vi "controlContinousBkwd.vi"(7 "Set":bool, 8 "error in":errorcluster, 9 "continous BWD in":bool=TRUE, 10 "axis in":u8, 11 "connection ID":i32) -> (0 "error out":errorcluster, 1 "continous BWD out":bool=TRUE, 2 "axis out":u8, 3 "connection ID":i32)   [LabVIEW 2016]
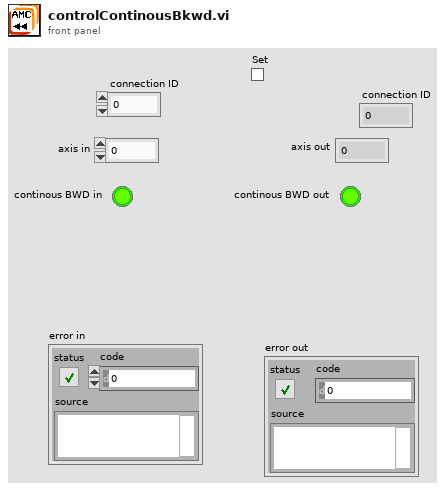
[diagram p1: front panel]
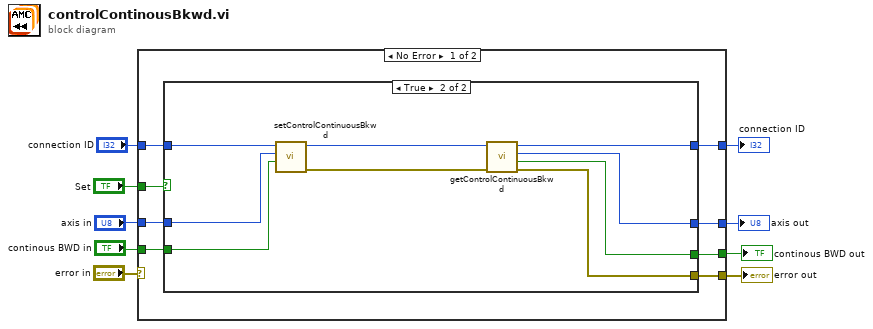
[diagram p0: block diagram]
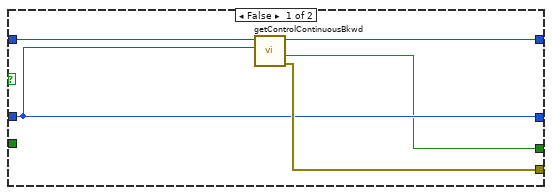
[diagram p2: hidden frame]
diagram:
  n1 = case shown="No Error" "error in" {
    selector: "error in" -> [_ w35]
    tunnel: "axis in" -> [w15 w33]
    tunnel: [w10 w35] -> w8
    tunnel: [w12 w33] -> w7
    tunnel: "Set" -> [w16 _]
    tunnel: [w11 w34] -> w5
    tunnel: "continous BWD in" -> [w14 w34]
    tunnel: [w13 w32] -> w3
    tunnel: "connection ID" -> [w17 w32]
    frame No Error {
      n2 = case shown="True" w16 {
        tunnel: [w21 w27] -> w13
        tunnel: w17 -> [w22 w31]
        tunnel: w15 -> [w19 w29]
        tunnel: [w19 w23] -> w12
        tunnel: [w18 w24] -> w11
        tunnel: [w20 w25] -> w10
        tunnel: w14 -> [_ w30]
        frame False {
          n3 = call "getControlContinuousBkwd.vi"("axis"=w19, "connection ID"=w22) -> ("error out"=w20:errorcluster, "enabled"=w18:bool, "connection ID"=w21:i32)  [unwired: 6 in, 1 out]
        }
        frame True {
          n4 = call "setControlContinuousBkwd.vi"("enable"=w30, "axis"=w29, "connection ID"=w31) -> ("error out"=w26:errorcluster, "connection ID"=w28:i32)  [unwired: 6 in, 1 out]
          n5 = call "getControlContinuousBkwd.vi"("error in"=w26, "connection ID"=w28) -> ("error out"=w25:errorcluster, "enabled"=w24:bool, "axis_out"=w23:i32, "connection ID"=w27:i32)  [unwired: 6 in]
        }
      }
    }
    frame Error {
    }
  }
  "error out" <- w8
  "axis out" <- w7
  "continous BWD out" <- w5
  "connection ID" <- w3
